vi "Launcher.vi"() -> ()   [LabVIEW 2021, in "Echo Reply Test With Server Manager.lvlib"]
uses:
  Echo Reply Test With Server Manager.lvlib
  WebSocket Actor/WebSocket Connection/Keepalive.ctl
  WS Test Server Subscriber/WS Test Server Subscriber.lvclass
  C:/Program Files/National Instruments/LabVIEW 2021/vi.lib/ActorFramework/Actor/Actor.lvclass
  WebSocket Actor/WebSocket Server Manager/WebSocket Server Manager.lvclass
  WebSocket Actor/WebSocket Server Manager/WebSocket Server Manager.lvclass/WebSocket Server Manager.ctl
  WS Test Server Subscriber/WS Test Server Subscriber.lvclass/WS Test Server Subscriber.ctl
  WS Test Client Subscriber/WS Test Client Subscriber.lvclass
  WS Test Client Subscriber/WS Test Client Subscriber.lvclass/WS Test Client Subscriber.ctl
  <vilib>/ActorFramework/Message Enqueuer/Message Enqueuer.lvclass/Message Enqueuer.ctl
  WS Test Client Subscriber/Write Keepalive.vi
  WebSocket Actor/WebSocket Server Manager/Write Keepalive.vi
  WS Test Server Subscriber/properties/Write WebSocket Server Manager Enqueuer.vi
  <vilib>/ActorFramework/Message Enqueuer/Enqueue.vi
  <vilib>/ActorFramework/Stop Msg/Stop Msg.lvclass
  C:/Program Files/National Instruments/LabVIEW 2021/vi.lib/ActorFramework/Message/Message.lvclass
  <vilib>/Utility/LVClass/Get LV Class Name.vi
  <resource>/AFDebug/Generate Trace for Message.vi
  <vilib>/ActorFramework/Message Priority Queue/Priority Enqueue.vi
  <vilib>/ActorFramework/Actor/Actor.lvclass
  <userlib>/_OpenG.lib/time/time.llb/openg_time.lvlib
  <userlib>/_OpenG.lib/error/error.llb/openg_error.lvlib
  WebSocket Actor/WebSocket Connection/WebSocket Connection.lvclass
panel:
  in  "Keepalive":T1={"Enabled"=TRUE, "Ping Interval (ms)"=25000, "Ping Timeout (ms)"=20000}
  in  "Stop Actors":bool
  in  "Number of Clients":i32=3
  out "error out":errorcluster
  # "In this example we will use the Server Manager Actor Infrastructure to launch a WebSocket server and we will illustrate a bidirectional communication between the WebSocket server and clients. \nWe launch one server that will define the /echo/ service. Then a user selectable number of clients can be launched. From such clients messages to the servers can be sent on the specified service. The server will echo back the message to the specific client. The server can broadcast messages to the clients. One can choose to send a series of messages at a certain time frequency. \nInstructions to execute the example;\n1. Run this VI\n2. Wait that the Server and Client GUI appear\n3. use the GUIs to exchange messages\n4. Stop the actors from this VI"
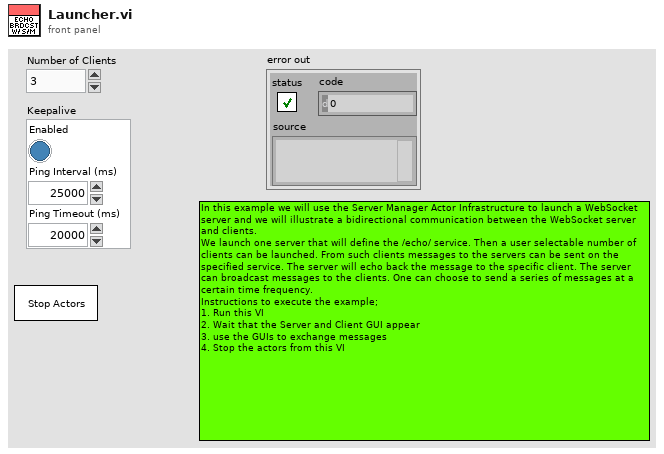
[diagram p1: front panel]
types:
  T1 = typedef "WebSocket Actors.lvlib/WebSocket Connection.lvclass/Keepalive.ctl" = cluster{"Enabled":bool, "Ping Interval (ms)":u32, "Ping Timeout (ms)":u32}
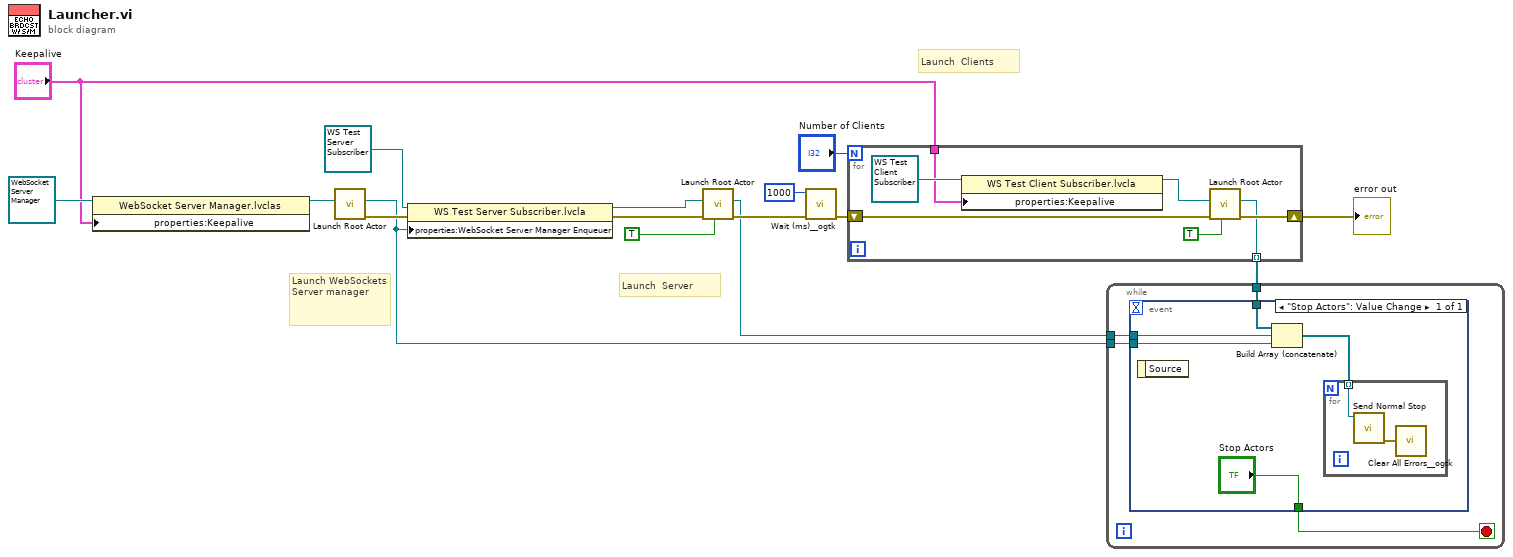
[diagram p0: block diagram]
diagram:
  # "Launch  Clients"
  # "Launch  Server"
  # "Launch WebSockets Server manager"
  n1 = property class="WebSocket Server Manager.lvclas"(reference=refnum<class "WebSocket Server Manager.lvclass"> refnum ("WebSocket Actors.lvlib:WebSocket Server Manager.lvclass"), "properties:Keepalive"="Keepalive") -> (reference out=w2:refnum<class "WebSocket Server Manager.lvclass">)  [unwired: 1 in, 1 out]
  n2 = call <vilib>:"Launch Root Actor.vi"("Actor"=w2) -> ("error out"=w10:errorcluster, "Actor's Enqueuer"=w6:refnum<class "Message Enqueuer.lvclass">)  [unwired: 9 in]
  n3 = property class="WS Test Server Subscriber.lvcla"(reference=refnum<class "WS Test Server Subscriber.lvclass"> refnum ("WS Full LabVIEW Test.lvlib:WS Test Server.lvclass"), error in=w10, "properties:WebSocket Server Manager Enqueuer"=w6) -> (reference out=w11:refnum<class "WS Test Server Subscriber.lvclass">, error out=w4:errorcluster)
  n4 = call <vilib>:"Launch Root Actor.vi"("Open Actor Core front panel? (F)"=TRUE, "error in (no error)"=w4, "Actor"=w11) -> ("error out"=w14:errorcluster, "Actor's Enqueuer"=w5:refnum<class "Message Enqueuer.lvclass">)  [unwired: 7 in]
  n5 = call <userlib>:"Wait (ms)__ogtk.vi"("error in (no error)"=w14, "milliseconds to wait"=u32 1000) -> ("error out"=w9:errorcluster)  [unwired: 8 in, 1 out]
  n6 = for {
    N: "Number of Clients" -> [_]
    shift-right: [w20] -> w13
    shift-left: w9 -> [w21]
    tunnel: [w19] -> w3 mode=indexing
    tunnel: "Keepalive" -> [w17]
    n7 = property class="WS Test Client Subscriber.lvcla"(reference=refnum<class "WS Test Client Subscriber.lvclass"> refnum ("WS Full LabVIEW Test.lvlib:WS Test Client.lvclass"), "properties:Keepalive"=w17) -> (reference out=w18:refnum<class "WS Test Client Subscriber.lvclass">)  [unwired: 1 in, 1 out]
    n8 = call <vilib>:"Launch Root Actor.vi"("Open Actor Core front panel? (F)"=TRUE, "error in (no error)"=w21, "Actor"=w18) -> ("error out"=w20:errorcluster, "Actor's Enqueuer"=w19:refnum<class "Message Enqueuer.lvclass">)  [unwired: 7 in]
  }
  "error out" <- w13
  n9 = while {
    tunnel: w6 -> [w27]
    tunnel: w5 -> [w25]
    tunnel: w3 -> [w24]
    stop <- w26 stop-if-true
    n10 = event shown="[0] \"Stop Actors\": Value Change" {
      selector: _ -> [_]
      dyn-events: _ -> [_]
      timeout: _ -> [_]
      tunnel: w27 -> [w32]
      tunnel: ["Stop Actors"] -> w26
      tunnel: w25 -> [w29]
      tunnel: w24 -> [w28]
      event "Stop Actors": Value Change {
        n11 = event-data() -> ()  [unwired: 1 in, 1 out]
        n12 = Build Array (concatenate)(w28, w29, w32) -> (w30:refnum<class "Message Enqueuer.lvclass">[])
        n13 = for {
          tunnel: w30 -> [w34] mode=indexing
          n14 = call <vilib>:"Send Normal Stop.vi"("Message Enqueuer"=w34) -> ("error out"=w33:errorcluster)  [unwired: 10 in]
          n15 = call <userlib>:"Clear All Errors__ogtk.vi"("Error In"=w33) -> ()  [unwired: 3 in, 1 out]
        }
      }
    }
  }
